vi "Meas Result Export.vi"(8 "error in":errorcluster, 11 "result":T1) -> (0 "error out":errorcluster)   [LabVIEW 2013]
doc: "Generates simple report to XLS. Excel must be installed!"
uses:
  Meas Results.ctl
  bridge/Bridge Frequency Readings Data.ctl
  drivers/TWM client/Meas Proc QWTB Spectrum Data.ctl
  Meas Results Sweep Data Uncertainty Mode.ctl
  <vilib>/Utility/miscctls.llb/LVRowAndColumnTypeDef.ctl
panel:
  in  "btn export":bool
  out "table":string[][](table) caption="Results"
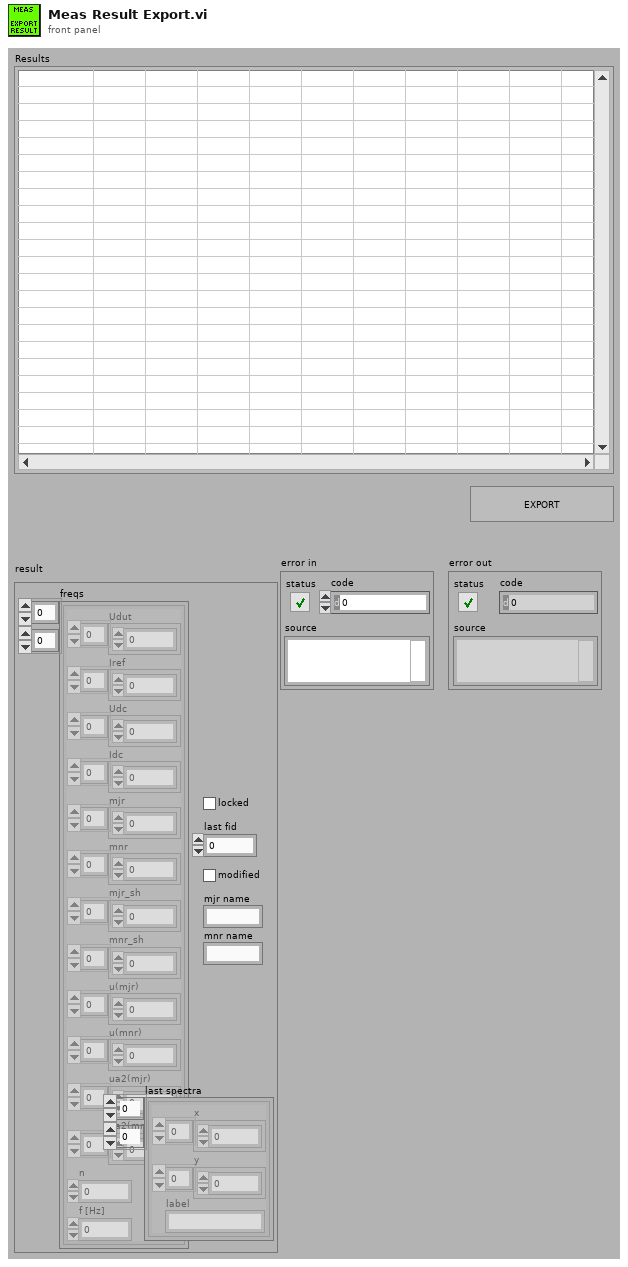
[diagram p1: front panel]
types:
  T1 = typedef "Meas Results.ctl" = cluster{"freqs":T2[][], "locked":bool, "last fid":i32, "modified":bool, "mjr name":string, "mnr name":string, "last spectra":T3[][]}
  T2 = typedef "Bridge Frequency Readings Data.ctl" = cluster{"Udut":dbl[], "Iref":dbl[], "Udc":dbl[], "Idc":dbl[], "mjr":dbl[], "mnr":dbl[], "mjr_sh":dbl[], "mnr_sh":dbl[], "u(mjr)":dbl[], "u(mnr)":dbl[], "ua2(mjr)":dbl[], "ua2(mnr)":dbl[], "n":i32, "f [Hz]":dbl}
  T3 = typedef "Meas Proc QWTB Spectrum Data.ctl" = cluster{"x":sgl[], "y":sgl[], "label":string}
  T4 = typedef "Meas Results Sweep Data Uncertainty Mode.ctl" = enum16{"ua(y)", "ua(y) (p=95%)", "uc(y) (p=95%)"}
  T5 = typedef "LVRowAndColumnTypeDef.ctl" = cluster{"Row":i32, "Column":i32}
  T6 = typedef "Meas Results Sweep Data.ctl" = cluster{"Udut":dbl[], "Iref":dbl[], "Udc":dbl[], "Idc":dbl[], "mjr":dbl[], "mnr":dbl[], "mjr_sh":dbl[], "mnr_sh":dbl[], "f [Hz]":dbl[]}
  T7 = typedef "Meas Quantity Names.ctl" = cluster{"mjr name":string, "mnr name":string, "mjr unit":string, "mnr unit":string, "mjr full":string, "mnr full":string}
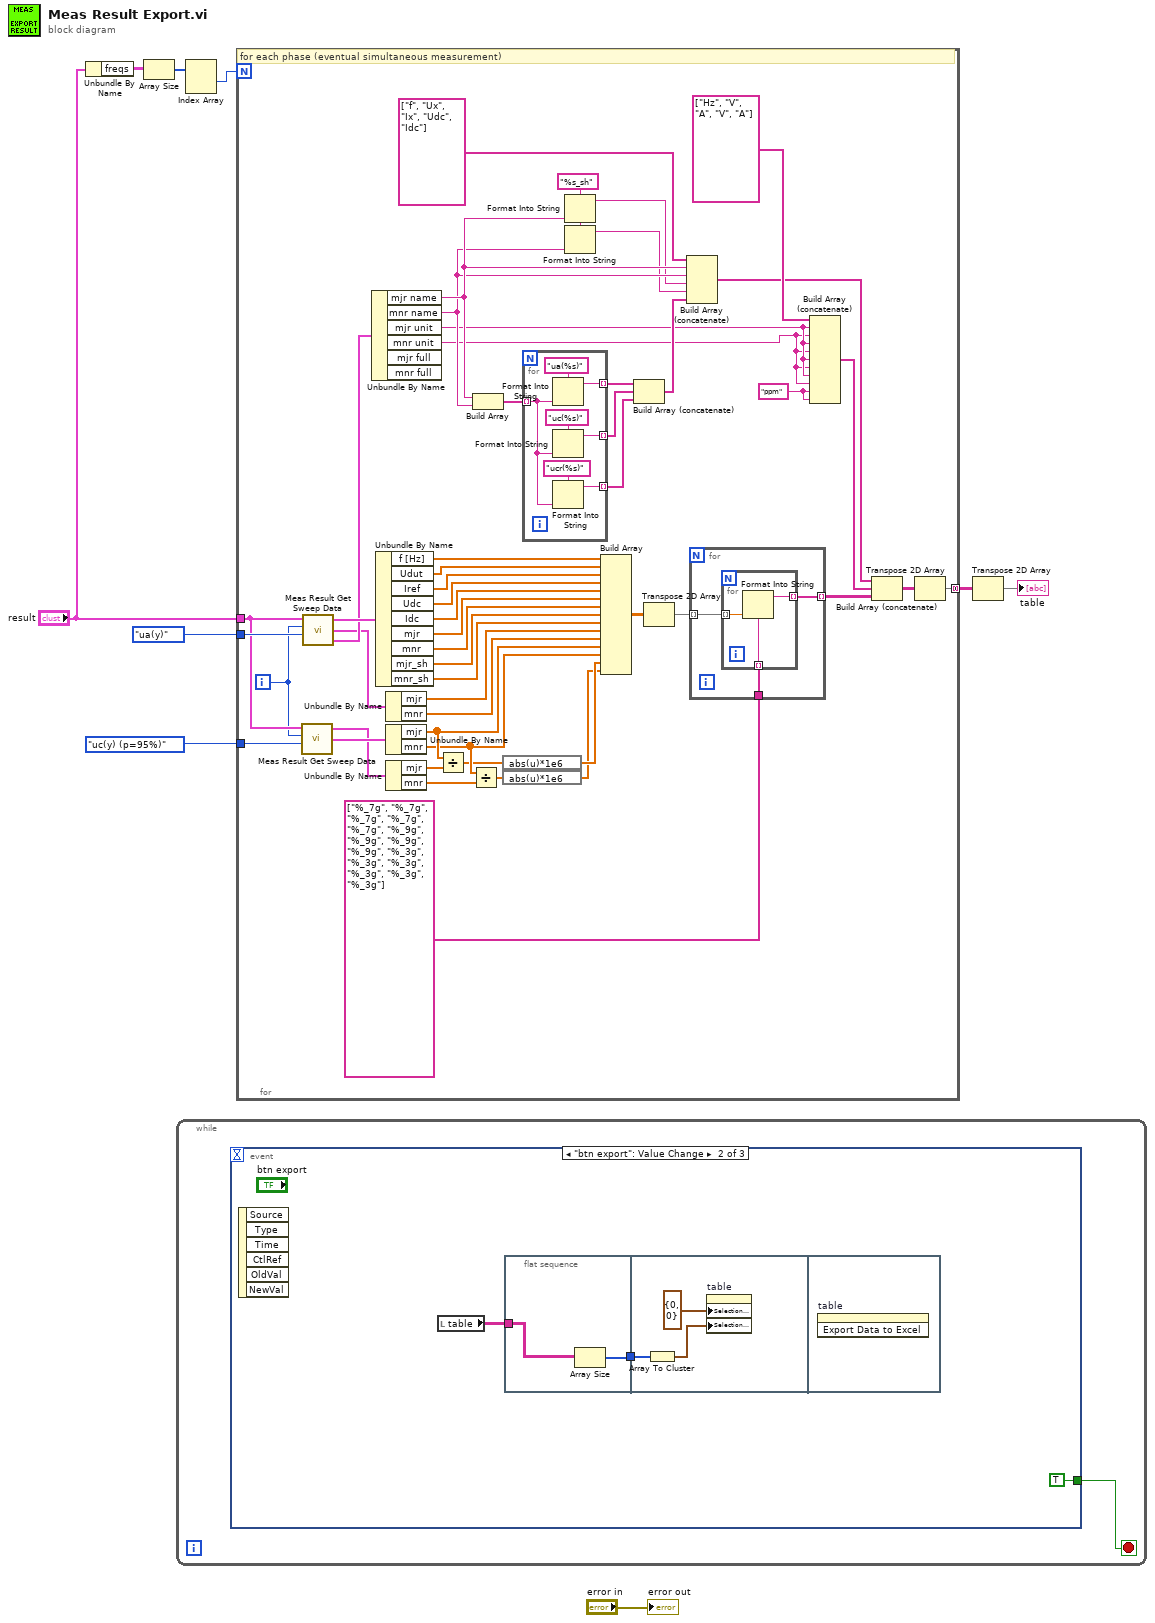
[diagram p0: block diagram]
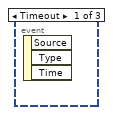
[diagram p2: hidden frame]
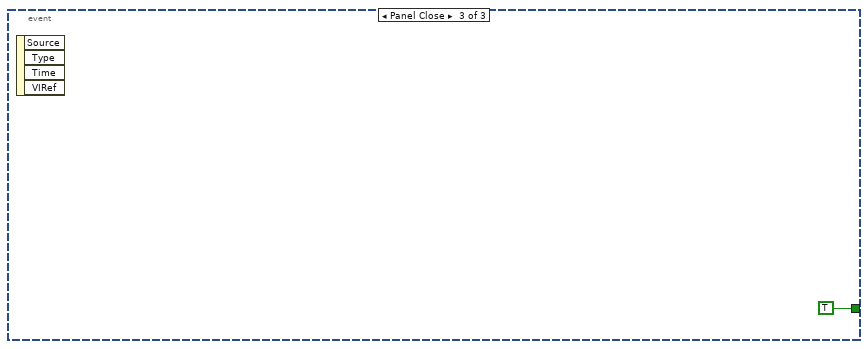
[diagram p3: hidden frame]
diagram:
  n1 = Unbundle By Name("result") -> ("freqs"=w3:T2[][])
  n2 = Array Size(array=w3) -> (size(s)=w2:i32[])
  n3 = while {
    stop <- w10 stop-if-true
    n4 = event shown="[1] \"btn export\": Value Change" {
      selector: _ -> [_ _ _]
      dyn-events: _ -> [_ _ _]
      timeout: _ -> [_ _ _]
      tunnel: [_ TRUE TRUE] -> w10
      event Timeout {
        n5 = event-data() -> ()  [unwired: 1 in, 3 out]
      }
      event "btn export": Value Change {
        n6 = event-data() -> ()  [unwired: 1 in, 6 out]
        n7 = local read "table"() -> (w12:string[][])
        n8 = flat-sequence {
          tunnel: w12 -> [w15]
          tunnel: [w14] -> w13
          tunnel: w13 -> [w17]
          frame #0 {
            n9 = Array Size(array=w15) -> (size(s)=w14:i32[])
          }
          frame #1 {
            n10 = Array To Cluster(array=w17) -> (cluster=w16:cluster{"[0]":i32, "[1]":i32})
            n11 = property on="table" class="Tbl (strict)"("Selection Start"=T5 {"Row"=0, "Column"=0}, "Selection Size"=w16) -> ()  [unwired: 2 in, 2 out]
          }
          frame #2 {
            n12 = invoke on="table" class="Tbl (strict)" method="Export Data to Excel"() -> ()  [unwired: 3 in, 3 out]
          }
        }
      }
      event Panel Close {
        n13 = event-data() -> ()  [unwired: 1 in, 4 out]
      }
    }
  }
  n14 = Index Array(array=w2) -> (element #1=w1:i32)  [unwired: 2 in, 1 out]
  n15 = for {
    N: w1 -> [_]
    tunnel: [w20] -> w8 mode=concatenating
    tunnel: Meas_Results_Sweep_Data_Uncertainty_Mode."ua(y)" ("uncertainty mode") -> [w51]
    tunnel: "result" -> [w50]
    tunnel: Meas_Results_Sweep_Data_Uncertainty_Mode."uc(y) (p=95%)" ("uncertainty mode") -> [w49]
    i -> [w21]
    w23 = "ppm" ("element")
    w39 = "%s_sh" ("format string")
    # "for each phase (eventual simultaneous measurement)"
    n16 = call "Meas Result Get Sweep Data.vi"("uncertainty mode"=w49, "phase index (default: 0)"=w21, "result"=w50) -> ("unc(data)"=w48:T6, "data"=w32:T6)  [unwired: 1 in, 1 out]
    n17 = call "Meas Result Get Sweep Data.vi"("uncertainty mode"=w51, "phase index (default: 0)"=w21, "result"=w50) -> ("quantities"=w69:T7, "unc(data)"=w52:T6, "data"=w70:T6)  [unwired: 1 in]
    n18 = Unbundle By Name(w69) -> ("mjr name"=w38:string, "mnr name"=w37:string, "mjr unit"=w34:string, "mnr unit"=w33:string)  [unwired: 2 out]
    n19 = Unbundle By Name(w70) -> ("f [Hz]"=w67:dbl[], "Udut"=w66:dbl[], "Iref"=w65:dbl[], "Udc"=w64:dbl[], "Idc"=w63:dbl[], "mjr"=w62:dbl[], "mnr"=w61:dbl[], "mjr_sh"=w41:dbl[], "mnr_sh"=w40:dbl[])
    n20 = Unbundle By Name(w52) -> ("mjr"=w47:dbl[], "mnr"=w46:dbl[])
    n21 = Unbundle By Name(w48) -> ("mjr"=w31:dbl[], "mnr"=w28:dbl[])
    n22 = Unbundle By Name(w32) -> ("mjr"=w30:dbl[], "mnr"=w29:dbl[])
    n23 = Divide(x=w31, y=w30) -> (x/y=w26:dbl[])
    n24 = Divide(x=w28, y=w29) -> (x/y=w27:dbl[])
    n25 = Build Array(w38, w37) -> (w45:string[])
    n26 = expression code="abs(u)*1e6"(w26) -> (w25:dbl[])
    n27 = expression code="abs(u)*1e6"(w27) -> (w24:dbl[])
    n28 = for {
      tunnel: w45 -> [w72] mode=indexing
      tunnel: [w75] -> w44 mode=indexing
      tunnel: [w74] -> w43 mode=indexing
      tunnel: [w71] -> w22 mode=indexing
      n29 = Format Into String(format string="ua(%s)", w72) -> (resulting string=w75:string)  [unwired: 2 in, 1 out]
      n30 = Format Into String(format string="uc(%s)", w72) -> (resulting string=w74:string)  [unwired: 2 in, 1 out]
      n31 = Format Into String(format string="ucr(%s)", w72) -> (resulting string=w71:string)  [unwired: 2 in, 1 out]
    }
    n32 = Format Into String(format string=w39, w38) -> (resulting string=w36:string)  [unwired: 2 in, 1 out]
    n33 = Format Into String(format string=w39, w37) -> (resulting string=w35:string)  [unwired: 2 in, 1 out]
    n34 = Build Array(w67, w66, w65, w64, w63, w62, w61, w41, w40, w47, w46, w31, w28, w25, w24) -> (w59:dbl[][])
    n35 = Build Array (concatenate)(w44, w43, w22) -> (w42:string[])
    n36 = Transpose 2D Array(2D array=w59) -> (transposed array=w58:dbl[][])
    n37 = Build Array (concatenate)(string[] ["f", "Ux", "Ix", "Udc", "Idc"], w38, w37, w36, w35, w42) -> (w55:string[])
    n38 = for {
      tunnel: w58 -> [w79] mode=indexing
      tunnel: string[] ["%_7g", "%_7g", "%_7g", "%_7g", "%_7g", "%_9g", "%_9g", "%_9g", "%_9g", "%_3g", "%_3g", "%_3g", "%_3g", "%_3g", "%_3g"] -> [w80]
      tunnel: [w78] -> w56 mode=indexing
      n39 = for {
        tunnel: w80 -> [w82] mode=indexing
        tunnel: w79 -> [w83] mode=indexing
        tunnel: [w81] -> w78 mode=indexing
        n40 = Format Into String(format string=w82, w83) -> (resulting string=w81:string)  [unwired: 2 in, 1 out]
      }
    }
    n41 = Build Array (concatenate)(string[] ["Hz", "V", "A", "V", "A"], w34, w33, w34, w33, w34, w33, w34, w33, w23, w23) -> (w54:string[])
    n42 = Build Array (concatenate)(w55, w54, w56) -> (w53:string[][])
    n43 = Transpose 2D Array(2D array=w53) -> (transposed array=w20:string[][])
  }
  n44 = Transpose 2D Array(2D array=w8) -> (transposed array=→"table":string[][])
  "error out" <- "error in"
